vi "ENC.vi"(8 "PWM.MAX":u16, 9 "PWM.CMP":u16, 10 "PWM.CNFG":u8 format="%08b", 11 "PWM.CS":u8) -> (3 "PWM.CNTR":u16)   [LabVIEW 2017]
uses:
  <vilib>/rvi/eio/common/nirviEmuTemplateMethod_errors.vi
  <vilib>/eio/EIOMethodNode/EIOMethodNode.xnode
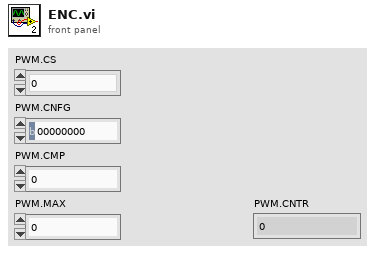
[diagram p1: front panel]
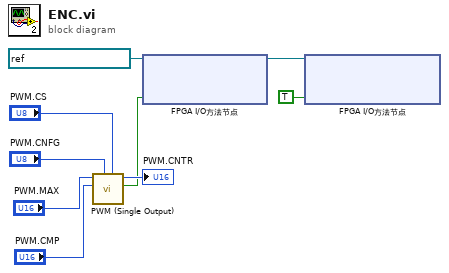
[diagram p0: block diagram]
diagram:
  n1 = call "PWM (Single Output).vi"("Clock Select"="PWM.CS", "Counter Control"="PWM.CNFG", "Output Compare Value"="PWM.CMP", "Max Counter Value"="PWM.MAX") -> ("Output"=w3:bool, "Counter Value"=→"PWM.CNTR":u16)  [unwired: 6 in]
  n2 = xnode "FPGA I/O方法节点"("FPGA I/O In"=refnum<k21> "ConnectorA/DIO8" ("DIO Refnum"), "Data"=w3) -> ("FPGA I/O Out"=w1:refnum<k21>)
  n3 = xnode "FPGA I/O方法节点"("FPGA I/O In"=w1, "Enable"=TRUE ("t")) -> ()  [unwired: 1 out]
